vi "LangmuirProbe-V-I-processing.vi"() -> ()   [LabVIEW 2014]
uses:
  subvi/myInteger.ctl
  <vilib>/Utility/miscctls.llb/LVPositionTypeDef.ctl
  <vilib>/Analysis/baseanly.llb/Mean (DBL).vi
  <vilib>/Analysis/3filter.llb/Savitzky-Golay Filter (DBL).vi
  <vilib>/Waveform/WDTOps.llb/WDT Waveform Duration DBL.vi
  <vilib>/Utility/file.llb/Read From Spreadsheet File (string).vi
  <vilib>/Utility/file.llb/Write To Spreadsheet File (string).vi
  <vilib>/Waveform/WDTOps.llb/WDT Get Waveform Subset DBL.vi
  <vilib>/measure/mascope.llb/Amplitude and Levels 1 chan.vi
  <vilib>/measure/NI_MAPro.lvlib
  <vilib>/Analysis/NI_AALBase.lvlib
panel:
  in  "zero drift control":T1={"start zero, ms"=1.0, "duration of zero,ms"=1.0, "'0',\nms"=FALSE} {"start zero, ms" min=0.15000000000000002 max=74.85000000000001; "duration of zero,ms" min=0.15000000000000002 max=74.85000000000001}
  in  "Cursor":bool
  in  "data info template":T2={"data path"="", "ADCintercadr_s"=1.0, "data info"={"use or not *.info.txt?"=0, "probe name"="NaN", "signal type"="NaN", "Unit"="NaN", "variable"="NaN", "attenuation factor"=1.0, "amplification factor"=1.0, "extracoef#1"=1.0, "extracoef#2"=1.0, "U cascade, kV"="NaN", "probe area, cm2"=1.0, "plasma, a.m.u."=1.0}, "channel_name"="", "channels_in_file"=0}
  in  "Boolean":bool
  out "saw biasing,adc":dbl format="%.3g"
  in  "sinchrY":bool
  in  "legend":bool
  in  "X axis":u16(ring)=1 items=["index", "time"]
  in  "êÃö":dbl=625.0
  in  "Vsmooth":bool
  in  "polyn.order V":i32=1 min=1
  in  "side points V":i32=2 min=2
  in  "I smooth":bool
  in  "polynomial order I":i32=1 min=1
  in  "side points I":i32=2 min=2
  in  "data select":T4={"V"=1, "I"=1, " V - \"noise\""=0, "I - \"noise\""=0, "1\"0\""=0.0, "2\"0\""=0.0, "3\"0\""=0.0, "4\"0\""=0.0, "Numeric"=0, "Numeric 2"=0, "Numeric 3"=0, "Numeric 4"=0, "U-nois subtr."=FALSE, "I-nois subtr."=FALSE} {"4\"0\"" format="%.4g"; "3\"0\"" format="%.4f"; "2\"0\"" format="%.4f"; "1\"0\"" format="%.4f"; "I - \"noise\"" items=["***", "11_05_54#1\\11_11_08", "11_05_54#2\\11_11_08", "11_05_54#3\\11_11_08", "11_05_54#4\\11_11_08", "11_05_54#5\\11_11_08", "11_05_54#6\\11_11_08", "11_05_54#7\\11_11_08", "11_05_54#8\\11_11_08", "11_05_54#9\\11_11_08", "11_05_54#10\\11_11_08", "11_05_54#11\\11_11_08", "11_05_54#12\\11_11_08", "11_05_54#13\\11_11_08", "11_05_54#14\\11_11_08", "11_05_54#15\\11_11_08", "11_05_54#16\\11_11_08", "11_05_54#17\\11_11_08", "11_05_54#18\\11_11_08", "11_05_54#19\\11_11_08", "11_05_54#20\\11_11_08", "11_05_54#21\\11_11_08", "11_05_54#22\\11_11_08", "11_05_54#23\\11_11_08", "11_05_54#24\\11_11_08", "11_05_54#25\\11_11_08", "11_05_54#26\\11_11_08", "11_05_54#27\\11_11_08", "11_05_54#28\\11_11_08", "11_05_54#29\\11_11_08", "11_05_54#30\\11_11_08"]; "V - \"noise\"" items=["***", "11_05_54#1\\11_11_08", "11_05_54#2\\11_11_08", "11_05_54#3\\11_11_08", "11_05_54#4\\11_11_08", "11_05_54#5\\11_11_08", "11_05_54#6\\11_11_08", "11_05_54#7\\11_11_08", "11_05_54#8\\11_11_08", "11_05_54#9\\11_11_08", "11_05_54#10\\11_11_08", "11_05_54#11\\11_11_08", "11_05_54#12\\11_11_08", "11_05_54#13\\11_11_08", "11_05_54#14\\11_11_08", "11_05_54#15\\11_11_08", "11_05_54#16\\11_11_08", "11_05_54#17\\11_11_08", "11_05_54#18\\11_11_08", "11_05_54#19\\11_11_08", "11_05_54#20\\11_11_08", "11_05_54#21\\11_11_08", "11_05_54#22\\11_11_08", "11_05_54#23\\11_11_08", "11_05_54#24\\11_11_08", "11_05_54#25\\11_11_08", "11_05_54#26\\11_11_08", "11_05_54#27\\11_11_08", "11_05_54#28\\11_11_08", "11_05_54#29\\11_11_08", "11_05_54#30\\11_11_08"]; "I" items=["***", "11_05_54#1\\11_11_08", "11_05_54#2\\11_11_08", "11_05_54#3\\11_11_08", "11_05_54#4\\11_11_08", "11_05_54#5\\11_11_08", "11_05_54#6\\11_11_08", "11_05_54#7\\11_11_08", "11_05_54#8\\11_11_08", "11_05_54#9\\11_11_08", "11_05_54#10\\11_11_08", "11_05_54#11\\11_11_08", "11_05_54#12\\11_11_08", "11_05_54#13\\11_11_08", "11_05_54#14\\11_11_08", "11_05_54#15\\11_11_08", "11_05_54#16\\11_11_08", "11_05_54#17\\11_11_08", "11_05_54#18\\11_11_08", "11_05_54#19\\11_11_08", "11_05_54#20\\11_11_08", "11_05_54#21\\11_11_08", "11_05_54#22\\11_11_08", "11_05_54#23\\11_11_08", "11_05_54#24\\11_11_08", "11_05_54#25\\11_11_08", "11_05_54#26\\11_11_08", "11_05_54#27\\11_11_08", "11_05_54#28\\11_11_08", "11_05_54#29\\11_11_08", "11_05_54#30\\11_11_08"]; "V" items=["***", "11_05_54#1\\11_11_08", "11_05_54#2\\11_11_08", "11_05_54#3\\11_11_08", "11_05_54#4\\11_11_08", "11_05_54#5\\11_11_08", "11_05_54#6\\11_11_08", "11_05_54#7\\11_11_08", "11_05_54#8\\11_11_08", "11_05_54#9\\11_11_08", "11_05_54#10\\11_11_08", "11_05_54#11\\11_11_08", "11_05_54#12\\11_11_08", "11_05_54#13\\11_11_08", "11_05_54#14\\11_11_08", "11_05_54#15\\11_11_08", "11_05_54#16\\11_11_08", "11_05_54#17\\11_11_08", "11_05_54#18\\11_11_08", "11_05_54#19\\11_11_08", "11_05_54#20\\11_11_08", "11_05_54#21\\11_11_08", "11_05_54#22\\11_11_08", "11_05_54#23\\11_11_08", "11_05_54#24\\11_11_08", "11_05_54#25\\11_11_08", "11_05_54#26\\11_11_08", "11_05_54#27\\11_11_08", "11_05_54#28\\11_11_08", "11_05_54#29\\11_11_08", "11_05_54#30\\11_11_08"]}
  in  "plot color":T5={"color1"=43051, "color2"=393471, "color3"=13762815, "color4"=16722475}
  in  "cursor":bool
  in  "apply param.":bool
  out "Y":dbl=0.9225555555555554 format="%#.6f"
  out "X":dbl=0.04447201268742792 format="%#.7f"
  in  "param.input":bool
  in  "stop 2":bool
  in  "stop":bool
  out "data view":waveform(dbl)[](graph) caption="ADC data"
  in  "Tab Control":enum32{"Te&ne"}(tab)
  in  "show XY":bool
  in  "autoscale":bool=TRUE
  out "manual I-V source":string[][](table)=[["30", "-0.5118"], ["20", "0.38385"], ["10", "1.9619"], ["0", "2.60165"], ["-4", "2.3884"], ["-5", "2.8149"], ["-10", "2.85755"], ["-11", "3.19875"], ["-20", "3.2414"], ["-60", "4.05175"], ["-80", "4.1797"], ["-100", "3.96645"], ["-130", "4.265"]] caption="manual I-V inpu"
  in  "manual I-V input":string[][](table)=[["30", "-0.5118"], ["20", "0.38385"], ["10", "1.9619"], ["0", "2.60165"], ["-4", "2.3884"], ["-5", "2.8149"], ["-10", "2.85755"], ["-11", "3.19875"], ["-20", "3.2414"], ["-60", "4.05175"], ["-80", "4.1797"], ["-100", "3.96645"], ["-130", "4.265"]] caption="manual I-V inpu"
  in  "Fit scales":bool
  in  "show/hide table":bool
  in  "man. points":bool
  in  "del. points":bool
  in  "man.XY table":bool
  out "TeNe":cluster{cdb[]}[](graph)=[{[nan+0.474455i, nan+0.415499i, nan+0.873553i, 10.1+17.942145i, 10.3+20.809732i, 10.4+20.192076i, 10.7+20.192076i, 10.7+29.74605i, 10.7+24.903581i, 12.0+20.184913i, 12.0+1190171.81586i, 14.0+29.746054i]}, {[nan+48551830000.0i, nan+44679440000.0i, nan+41846650000.0i, 10.1+1606494000000.0i, 10.3+1406263000000.0i, 10.4+1449819000000.0i, 10.7+1288728000000.0i, 10.7+1769306000000.0i, 10.7+2116097000000.0i, 12.0+2004418000000.0i, 12.0+501530900000000.0i, 14.0+95067200000.0i]}]
  in  "manual coef. input":bool
  in  "manual param. input":T6={"R, ohm"=100.0, "saw bias., V"=180.0, "plasma, a.u.m."=1.0, "probe area, cm^2"=0.07, "position, etc."=13.999999999999996, "probe name"="VG8#1", "I amplif."=10.0, "saw bias., V(ADC)"=0.0} {"saw bias., V(ADC)" format="%#.6f"; "saw bias., V" min=1.0}
  in  "Limited by cursors":bool
  in  "Parameter Name      Parameter Guess        Fit?":T7={"parameter"="Te, eV", "Te_guess"=10.0, "Fit?"=TRUE} {"Te_guess" min=0.0}
  in  "Parameter Name      Parameter Guess        Fit? 3":T8={"parameter"="Vfl, V", "Vf_guess"=-10.0, "Fit?"=TRUE}
  in  "parameter                 manual            auto?":T9={"parameter"="Is, A", "Is_guess"=0.01, "Fit?"=TRUE}
  in  "save result":bool
  in  "processing":bool
  in  "show result":bool
  out "param.        manual.     auto?      auto             result":T10(array[cluster])=[{"parameter"="Is(mA)", "guess"=5.0, "Fit?"=TRUE, "best fit"=3.774695434023404, "result"=3.774695434023404}, {"parameter"="Vfl(V)", "guess"=0.0, "Fit?"=TRUE, "best fit"=-1.3923455769080333, "result"=-1.3923455769080333}, {"parameter"="Te(eV)", "guess"=3.0, "Fit?"=TRUE, "best fit"=1.9615172489090944, "result"=1.9615172489090944}] {"result" format="%#.6f"; "best fit" format="%#.6f"}
  out "density, cm^(-3)":dbl=24256512471.923824 format="%#.2e"
  out "Y":dbl format="%#.2g"
  out "X":dbl format="%#.2g"
  out "ln(I,I-bestfit)":cluster{cdb[]}[](graph)
  out "VI-fitgraph":cluster{cdb[]}[](graph)=[{[30.0-0.5118i, 20.0+0.38385i, 10.0+1.9619i, 0.0+2.60165i, -4.0+2.3884i, -5.0+2.8149i, -10.0+2.85755i, -11.0+3.19875i, -20.0+3.2414i, -60.0+4.05175i, -80.0+4.1797i, -100.0+3.96645i, -130.0+4.265i]}]
  out "result table":string[][](array[string])=[["                     file", "                 interval", "               probe name", "                 variable", "                  Is (mA)", "              Vfl (Volts)", "                  Te (eV)", "         density (cm**-3)"], ["                 10_36_46", "           t0.0373-0.0398", "                      NaN", "                      NaN", "                 3.715870", "                -0.124411", "                 0.474455", "             4.855183E+10"], ["                 10_10_55", "           t0.0152-0.0784", "                      NaN", "                      NaN", "                 3.200000", "                -0.087612", "                 0.415499", "             4.467944E+10"], ["                 10_12_10", "           t0.0272-0.0353", "                      NaN", "                      NaN", "                 4.345731", "                -0.052320", "                 0.873553", "             4.184665E+10"], ["                 10_45_04", "           t0.0235-0.0275", "                    VG8#1", "                10.100000", "                52.926325", "                -4.701742", "                17.942145", "             1.606494E+12"], ["                 10_45_04", "           t0.0235-0.0275", "                    VG8#1", "                10.300000", "                57.022652", "                -4.877215", "                20.809732", "             1.406263E+12"], ["                 10_45_04", "           t0.0235-0.0275", "                    VG8#1", "                10.400000", "                57.909756", "                -4.862004", "                20.192076", "             1.449819E+12"], ["                 10_45_04", "           t0.0235-0.0275", "                    VG8#1", "                10.700000", "                57.909756", "                -4.862004", "                20.192076", "             1.288728E+12"], ["                 10_45_04", "           t0.0235-0.0275", "                    VG8#1", "                10.700000", "                64.331903", "                -5.056201", "                29.746050", "             1.769306E+12"], ["                 10_45_04", "           t0.0235-0.0275", "                    VG8#1", "                10.700000", "                58.667018", "                -5.613754", "                24.903581", "             2.116097E+12"], ["                 10_45_04", "           t0.0235-0.0275", "                    VG8#1", "                12.000000", "                50.029859", "                -5.289460", "                20.184913", "             2.004418E+12"], ["                 10_45_04", "           t0.0235-0.0275", "                    VG8#1", "                12.000000", "           3039694.842475", "                -6.242550", "           1190171.815860", "             5.015309E+14"], ["                 10_45_04", "           t0.0235-0.0275", "                    VG8#1", "                14.000000", "                57.610661", "                -5.056201", "                29.746054", "             9.506720E+10"]]
  out "TeNe result":path=path "d:/_TeNe.txt"
  out "TeNe file":string="***"
  out "TeNe interval":string="t0.0216-0.0259"
  in  "press after parameters input":bool
  out "data info manual input sample":string[][](table)=[["11_00_19", "2", "VG1#1", "LP_biasing", "10.25", "1", "1", "162", "1", "5,6", "0.07", "1"], ["=", "4", "VG1#2", "LP_current", "10.25", "1", "1", "300", "1", "5,6", "0.07", "1"], ["11_00_44", "2", "VG1#1", "LP_biasing", "10.25", "1", "1", "162", "1", "5,6", "0.07", "1"], ["=", "4", "VG1#2", "LP_current", "10.25", "1", "1", "300", "1", "5,6", "0.07", "1"]]
  in  "data info manual input":string[][](table)=[["11_00_44", "2", "", "V", "10.25", "", "1", "162", "", "", "0.07", "1"], ["=", "4", "", "I", "10.25", "", "1", "300", "", "", "0.07", "1"], ["11_00_44", "2", "", "V", "10.25", "", "1", "162", "", "", "0.07", "1"], ["=", "4", "", "I", "10.25", "", "1", "300", "", "", "0.07", "1"], ["11_00_44", "2", "", "V", "10.25", "", "1", "162", "", "", "0.07", "1"], ["=", "4", "", "I", "10.25", "", "1", "300", "", "", "0.07", "1"]]
  out "source":T11={"data path"=["D:\\LCard\\ADC\\LPBPP\\30_09_15\\_0214_E-2010_4R235953#1", "D:\\LCard\\ADC\\LPBPP\\30_09_15\\_0214_E-2010_4R235953#2", "D:\\LCard\\ADC\\LPBPP\\30_09_15\\_0214_E-2010_4R235953#3"], "data"=[{"t0"=timestamp(0 s since 1904-01-01), "dt"=4e-07, "Y"=array[250000 elements], "attributes"=variant("info"=variant(cluster{"data path":string, "ADCcadrlength_s":dbl, "data info":cluster{"use or not *.info.txt?":i16, "probe name":string, "signal type":string, "Unit":string, "variable":string, "attenuation factor":dbl, "amplification factor":dbl, "extracoef#1":dbl, "extracoef#2":dbl, "U cascade, kV":string, "probe area, cm2":dbl, "plasma, a.m.u.":dbl}} {"data path"="D:\\LCard\\ADC\\LPBPP\\30_09_15\\_0214_E-2010_4R235953#1", "ADCcadrlength_s"=2500000.0, "data info"={"use or not *.info.txt?"=0, "probe name"="NaN", "signal type"="NaN", "Unit"="NaN", "variable"="NaN", "attenuation factor"=1.0, "amplification factor"=1.0, "extracoef#1"=1.0, "extracoef#2"=1.0, "U cascade, kV"="NaN", "probe area, cm2"=1.0, "plasma, a.m.u."=1.0}}))}, {"t0"=timestamp(1.3333333333330043e-07 s since 1904-01-01), "dt"=4e-07, "Y"=array[250000 elements], "attributes"=variant("info"=variant(cluster{"data path":string, "ADCcadrlength_s":dbl, "data info":cluster{"use or not *.info.txt?":i16, "probe name":string, "signal type":string, "Unit":string, "variable":string, "attenuation factor":dbl, "amplification factor":dbl, "extracoef#1":dbl, "extracoef#2":dbl, "U cascade, kV":string, "probe area, cm2":dbl, "plasma, a.m.u.":dbl}} {"data path"="D:\\LCard\\ADC\\LPBPP\\30_09_15\\_0214_E-2010_4R235953#2", "ADCcadrlength_s"=2500000.0, "data info"={"use or not *.info.txt?"=0, "probe name"="NaN", "signal type"="NaN", "Unit"="NaN", "variable"="NaN", "attenuation factor"=1.0, "amplification factor"=1.0, "extracoef#1"=1.0, "extracoef#2"=1.0, "U cascade, kV"="NaN", "probe area, cm2"=1.0, "plasma, a.m.u."=1.0}}))}, {"t0"=timestamp(2.666666666666551e-07 s since 1904-01-01), "dt"=4e-07, "Y"=array[250000 elements], "attributes"=variant("info"=variant(cluster{"data path":string, "ADCcadrlength_s":dbl, "data info":cluster{"use or not *.info.txt?":i16, "probe name":string, "signal type":string, "Unit":string, "variable":string, "attenuation factor":dbl, "amplification factor":dbl, "extracoef#1":dbl, "extracoef#2":dbl, "U cascade, kV":string, "probe area, cm2":dbl, "plasma, a.m.u.":dbl}} {"data path"="D:\\LCard\\ADC\\LPBPP\\30_09_15\\_0214_E-2010_4R235953#3", "ADCcadrlength_s"=2500000.0, "data info"={"use or not *.info.txt?"=0, "probe name"="NaN", "signal type"="NaN", "Unit"="NaN", "variable"="NaN", "attenuation factor"=1.0, "amplification factor"=1.0, "extracoef#1"=1.0, "extracoef#2"=1.0, "U cascade, kV"="NaN", "probe area, cm2"=1.0, "plasma, a.m.u."=1.0}}))}]}
  out "num-of-plots":i32=4
  out "data cut":T12={"data offset array"=[0.021598275434243176, 0.021598275434243176, 0.021598275434243176, 0.021598275434243176, 0.021598275434243176, 0.021598275434243176], "data cut array"=[{"t0"=timestamp(0.0215984 s since 1904-01-01), "dt"=4e-07, "Y"=array[10854 elements], "attributes"=variant("info"=variant(cluster{"data path":string, "ADCintercadr_s":dbl, "data info":cluster{"use or not *.info.txt?":i16, "probe name":string, "signal type":string, "Unit":string, "variable":string, "attenuation factor":dbl, "amplification factor":dbl, "extracoef#1":dbl, "extracoef#2":dbl, "U cascade, kV":string, "probe area, cm2":dbl, "plasma, a.m.u.":dbl}} {"data path"="***", "ADCintercadr_s"=2500000.0, "data info"={"use or not *.info.txt?"=0, "probe name"="NaN", "signal type"="NaN", "Unit"="NaN", "variable"="NaN", "attenuation factor"=1.0, "amplification factor"=1.0, "extracoef#1"=1.0, "extracoef#2"=1.0, "U cascade, kV"="NaN", "probe area, cm2"=1.0, "plasma, a.m.u."=1.0}}))}, {"t0"=timestamp(0.0215984 s since 1904-01-01), "dt"=4e-07, "Y"=array[10854 elements], "attributes"=variant("info"=variant(cluster{"data path":string, "ADCintercadr_s":dbl, "data info":cluster{"use or not *.info.txt?":i16, "probe name":string, "signal type":string, "Unit":string, "variable":string, "attenuation factor":dbl, "amplification factor":dbl, "extracoef#1":dbl, "extracoef#2":dbl, "U cascade, kV":string, "probe area, cm2":dbl, "plasma, a.m.u.":dbl}} {"data path"="***", "ADCintercadr_s"=2500000.0, "data info"={"use or not *.info.txt?"=0, "probe name"="NaN", "signal type"="NaN", "Unit"="NaN", "variable"="NaN", "attenuation factor"=1.0, "amplification factor"=1.0, "extracoef#1"=1.0, "extracoef#2"=1.0, "U cascade, kV"="NaN", "probe area, cm2"=1.0, "plasma, a.m.u."=1.0}}))}, {"t0"=timestamp(0.0215984 s since 1904-01-01), "dt"=4e-07, "Y"=array[10854 elements], "attributes"=variant("info"=variant(cluster{"data path":string, "ADCintercadr_s":dbl, "data info":cluster{"use or not *.info.txt?":i16, "probe name":string, "signal type":string, "Unit":string, "variable":string, "attenuation factor":dbl, "amplification factor":dbl, "extracoef#1":dbl, "extracoef#2":dbl, "U cascade, kV":string, "probe area, cm2":dbl, "plasma, a.m.u.":dbl}} {"data path"="***", "ADCintercadr_s"=2500000.0, "data info"={"use or not *.info.txt?"=0, "probe name"="NaN", "signal type"="NaN", "Unit"="NaN", "variable"="NaN", "attenuation factor"=1.0, "amplification factor"=1.0, "extracoef#1"=1.0, "extracoef#2"=1.0, "U cascade, kV"="NaN", "probe area, cm2"=1.0, "plasma, a.m.u."=1.0}}))}, {"t0"=timestamp(0.0215984 s since 1904-01-01), "dt"=4e-07, "Y"=array[10854 elements], "attributes"=variant("info"=variant(cluster{"data path":string, "ADCintercadr_s":dbl, "data info":cluster{"use or not *.info.txt?":i16, "probe name":string, "signal type":string, "Unit":string, "variable":string, "attenuation factor":dbl, "amplification factor":dbl, "extracoef#1":dbl, "extracoef#2":dbl, "U cascade, kV":string, "probe area, cm2":dbl, "plasma, a.m.u.":dbl}} {"data path"="***", "ADCintercadr_s"=2500000.0, "data info"={"use or not *.info.txt?"=0, "probe name"="NaN", "signal type"="NaN", "Unit"="NaN", "variable"="NaN", "attenuation factor"=1.0, "amplification factor"=1.0, "extracoef#1"=1.0, "extracoef#2"=1.0, "U cascade, kV"="NaN", "probe area, cm2"=1.0, "plasma, a.m.u."=1.0}}))}, {"t0"=timestamp(0.0215984 s since 1904-01-01), "dt"=4e-07, "Y"=array[10854 elements], "attributes"=variant("info"=variant(cluster{"data path":string, "ADCintercadr_s":dbl, "data info":cluster{"use or not *.info.txt?":i16, "probe name":string, "signal type":string, "Unit":string, "variable":string, "attenuation factor":dbl, "amplification factor":dbl, "extracoef#1":dbl, "extracoef#2":dbl, "U cascade, kV":string, "probe area, cm2":dbl, "plasma, a.m.u.":dbl}} {"data path"="***", "ADCintercadr_s"=2500000.0, "data info"={"use or not *.info.txt?"=0, "probe name"="NaN", "signal type"="NaN", "Unit"="NaN", "variable"="NaN", "attenuation factor"=1.0, "amplification factor"=1.0, "extracoef#1"=1.0, "extracoef#2"=1.0, "U cascade, kV"="NaN", "probe area, cm2"=1.0, "plasma, a.m.u."=1.0}}))}, {"t0"=timestamp(0.0215984 s since 1904-01-01), "dt"=4e-07, "Y"=array[10854 elements], "attributes"=variant("info"=variant(cluster{"data path":string, "ADCintercadr_s":dbl, "data info":cluster{"use or not *.info.txt?":i16, "probe name":string, "signal type":string, "Unit":string, "variable":string, "attenuation factor":dbl, "amplification factor":dbl, "extracoef#1":dbl, "extracoef#2":dbl, "U cascade, kV":string, "probe area, cm2":dbl, "plasma, a.m.u.":dbl}} {"data path"="***", "ADCintercadr_s"=2500000.0, "data info"={"use or not *.info.txt?"=0, "probe name"="NaN", "signal type"="NaN", "Unit"="NaN", "variable"="NaN", "attenuation factor"=1.0, "amplification factor"=1.0, "extracoef#1"=1.0, "extracoef#2"=1.0, "U cascade, kV"="NaN", "probe area, cm2"=1.0, "plasma, a.m.u."=1.0}}))}], "data lables"=["***=t0.0216-0.0259", "***=t0.0216-0.0259", "***=t0.0216-0.0259", "***=t0.0216-0.0259", "***=t0.0216-0.0259", "***=t0.0216-0.0259"], "short data lables"=["\\***=t0.0216-0.0259", "\\***=t0.0216-0.0259", "\\***=t0.0216-0.0259", "\\***=t0.0216-0.0259", "\\***=t0.0216-0.0259", "\\***=t0.0216-0.0259"]}
  # "ctr+\"click\" to add points !"
  # "set all parameters as close as possible\nto expected values !!!"
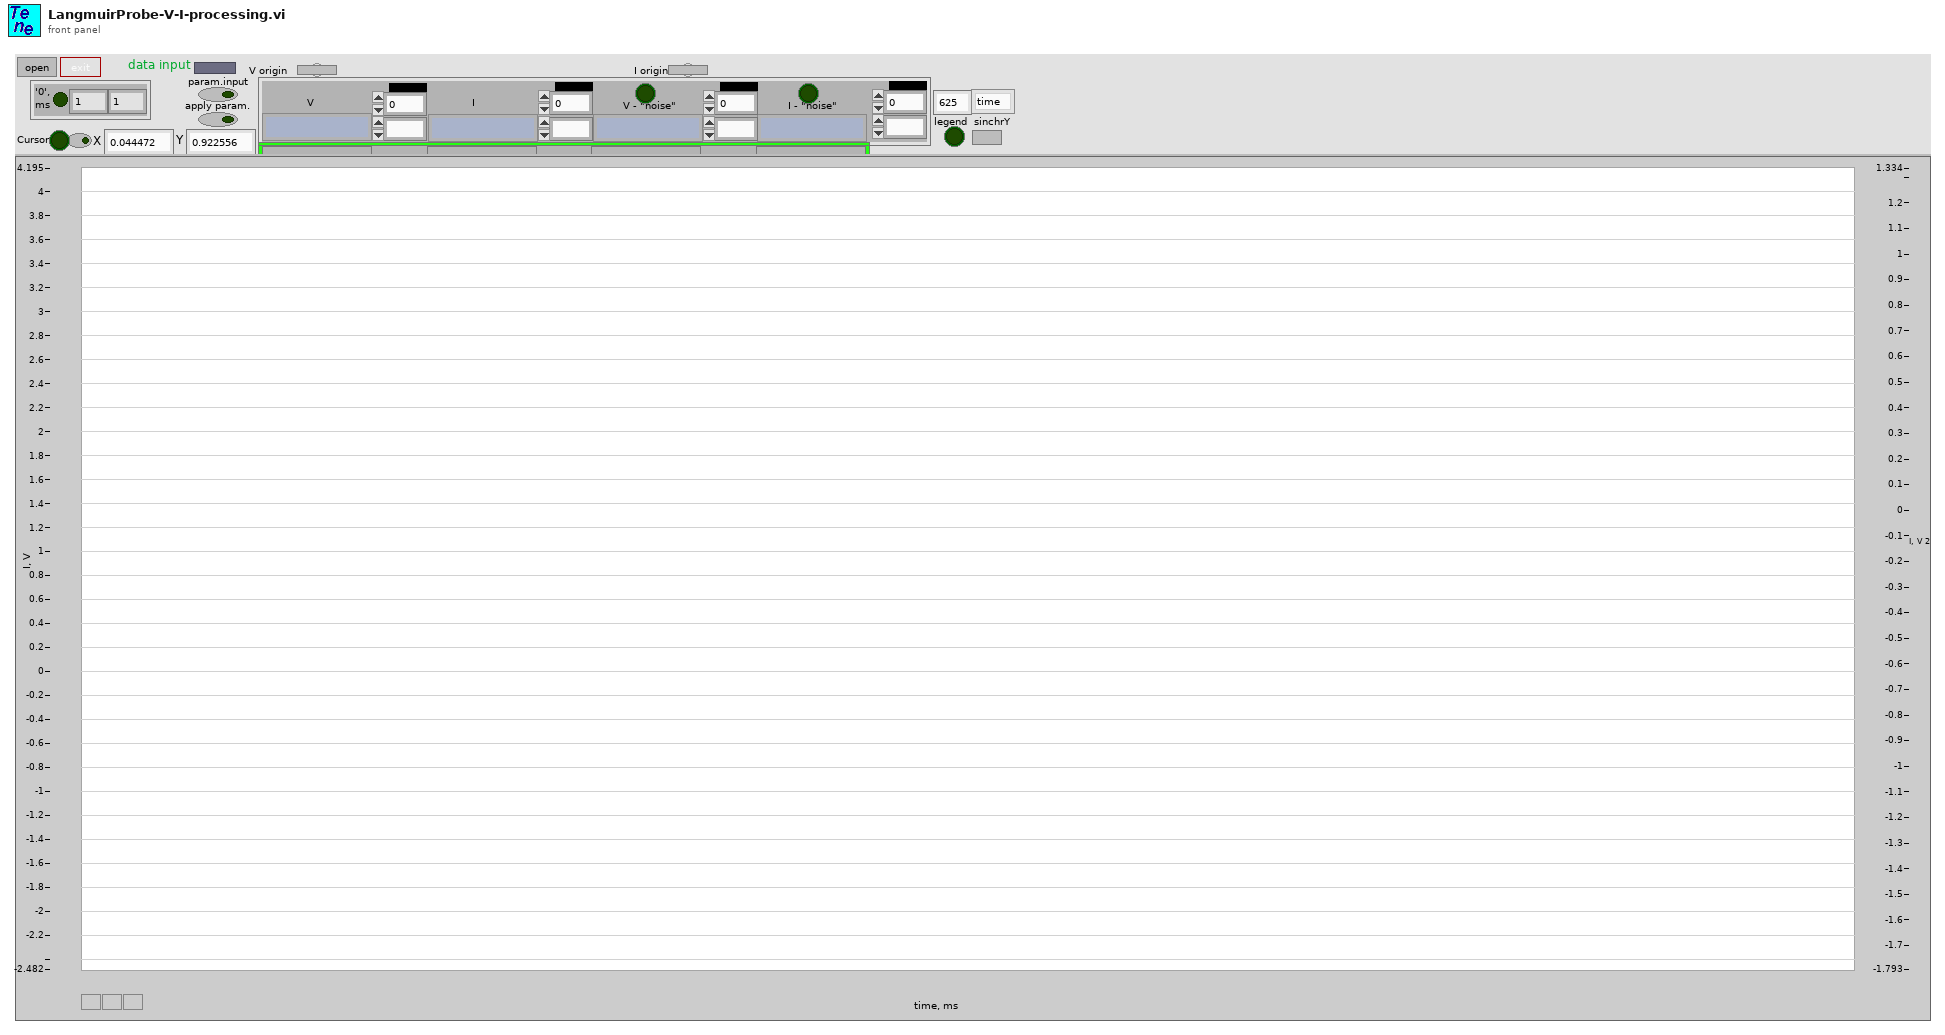
[diagram p1: front panel]
types:
  T1 = cluster{"start zero, ms":dbl, "duration of zero,ms":dbl, "'0',\nms":bool}
  T2 = cluster{"data path":string, "ADCintercadr_s":dbl, "data info":cluster{"use or not *.info.txt?":i16, "probe name":string, "signal type":string, "Unit":string, "variable":string, "attenuation factor":dbl, "amplification factor":dbl, "extracoef#1":dbl, "extracoef#2":dbl, "U cascade, kV":string, "probe area, cm2":dbl, "plasma, a.m.u.":dbl}, "channel_name":string, "channels_in_file":i32}
  T3 = typedef "myInteger.ctl" = i32
  T4 = cluster{"V":u16, "I":u16, " V - \"noise\"":u16, "I - \"noise\"":u16, "1\"0\"":dbl, "2\"0\"":dbl, "3\"0\"":dbl, "4\"0\"":dbl, "Numeric":T3, "Numeric 2":T3, "Numeric 3":T3, "Numeric 4":T3, "U-nois subtr.":bool, "I-nois subtr.":bool}
  T5 = cluster{"color1":u32, "color2":u32, "color3":u32, "color4":u32}
  T6 = cluster{"R, ohm":dbl, "saw bias., V":dbl, "plasma, a.u.m.":dbl, "probe area, cm^2":dbl, "position, etc.":dbl, "probe name":string, "I amplif.":dbl, "saw bias., V(ADC)":dbl}
  T7 = cluster{"parameter":string, "Te_guess":dbl, "Fit?":bool}
  T8 = cluster{"parameter":string, "Vf_guess":dbl, "Fit?":bool}
  T9 = cluster{"parameter":string, "Is_guess":dbl, "Fit?":bool}
  T10 = cluster{"parameter":string, "guess":dbl, "Fit?":bool, "best fit":dbl, "result":dbl}[]
  T11 = cluster{"data path":string[], "data":waveform(dbl)[]}
  T12 = cluster{"data offset array":dbl[], "data cut array":waveform(dbl)[], "data lables":string[], "short data lables":string[]}
  T13 = typedef "LVPositionTypeDef.ctl" = cluster{"Left":i32, "Top":i32}
  T14 = cluster{"method":enum32{"histogram", "peak", "auto select"}, "histogram size":i32, "histogram method":enum16{"mode"}, "reserved":dbl}
  T15 = cluster{"Name":string, "Color":u32, "Style":u8, "Point Style":u8, "Name Visible":bool, "Allow Drag":bool, "Cursor Mode":u32, "Plot":i32, "Index":i32, "Position":cluster{"X":dbl, "Y":dbl}, "X Scale":u32, "Y Scale":u32, "Watch Plots":i32[], "Watch All Plots":bool, "Plot Area":i32, "Label Offset":cluster{"X":dbl, "Y":dbl}}
  T16 = cluster{"V":u16, "I":u16, " V - \"noise\"":u16, "I - \"noise\"":u16}
  T17 = cluster{cluster{"V":u16, "I":u16, " V - \"noise\"":u16, "I - \"noise\"":u16}, "plot color":cluster{"color1":u32, "color2":u32, "color3":u32, "color4":u32}}
  T18 = typedef "LVRangeTypeDef.ctl" = cluster{"Minimum":dbl, "Maximum":dbl, "Increment":dbl, "Minor Increment":dbl, "Start":dbl}
  T19 = cluster{"use or not *.info.txt?":i16, "probe name":string, "signal type":string, "Unit":string, "variable":string, "attenuation factor":dbl, "amplification factor":dbl, "extracoef#1":dbl, "extracoef#2":dbl, "U cascade, kV":string, "probe area, cm2":dbl, "plasma, a.m.u.":dbl}
  T20 = typedef "LVPointDoubleTypeDef.ctl" = cluster{"Cursor X":dbl, "Cursor Y":dbl}
  T21 = typedef "LVCursorListTypeDef.ctl" = cluster{"Name":string, "Color":u32, "Style":u8, "Point Style":u8, "Name Visible":bool, "Allow Drag":bool, "Cursor Mode":u32, "Plot":i32, "Index":i32, "Position":cluster{"X":dbl, "Y":dbl}, "X Scale":u32, "Y Scale":u32, "Watch Plots":i32[], "Watch All Plots":bool, "Plot Area":i32, "Label Offset":cluster{"X":dbl, "Y":dbl}}[]
  T22 = enum8{"Enabled", "Disabled", "Disabled and Grayed Out"}
  T23 = cluster{"parameter":string, "guess":dbl, "Fit?":bool, "best fit":dbl, "result":dbl}
  T24 = typedef "LVPoint32TypeDef.ctl" = cluster{"Horizontal":i32, "Vertical":i32}
  T25 = cluster{"Shift":bool, "Ctrl":bool, "Alt":bool, "Cmd":bool, "Opt":bool}
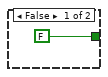
[diagram p3: hidden frame]
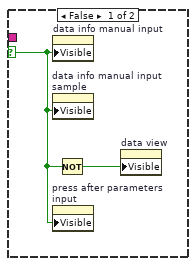
[diagram p5: hidden frame]
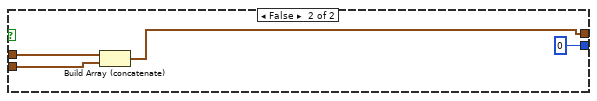
[diagram p9: hidden frame]
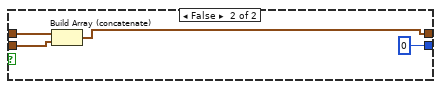
[diagram p10: hidden frame]
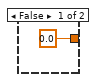
[diagram p11: hidden frame]
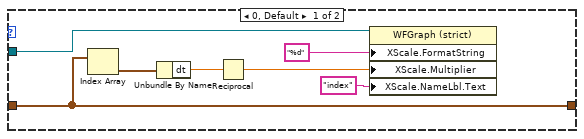
[diagram p13: hidden frame]
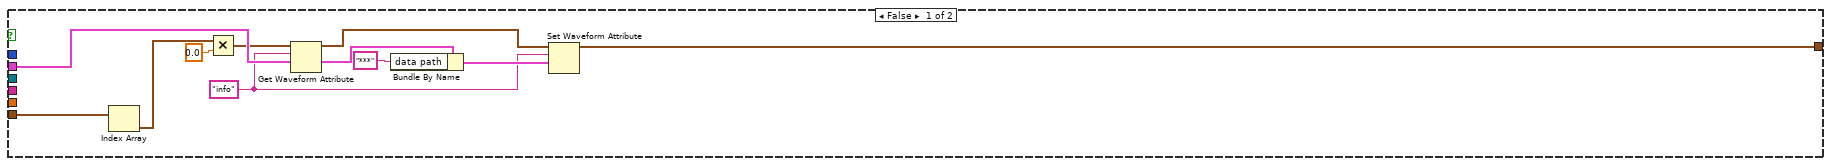
[diagram p14: hidden frame]
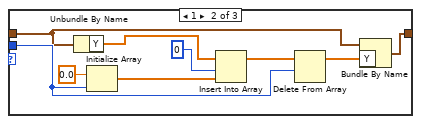
[diagram p16: hidden frame]
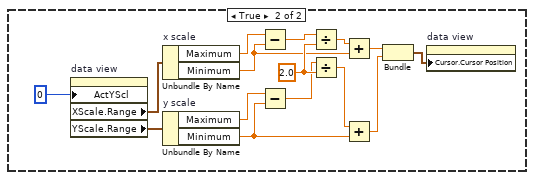
[diagram p18: hidden frame]
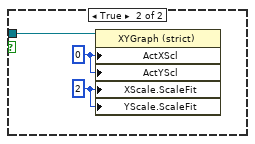
[diagram p20: hidden frame]
diagram:
  n1 = while {
    stop <- FALSE stop-if-true
    n2 = control-ref of="data info template"() -> (w5:refnum<vi>)
    n3 = call "DATAreader5.vi"("manual ADC rate, kHz"="êÃö", "data info template"=w5) -> ("error out"=w3:errorcluster, "source"=→"source":T11)  [unwired: 4 in, 4 out]
    n4 = invoke on="man.XY table" class="Bool (strict)" method="Reinit To Default"(error in=w3) -> (error out=w1:errorcluster)  [unwired: 2 in, 2 out]
    n5 = invoke on="processing" class="Bool (strict)" method="Reinit To Default"(error in=w1) -> (error out=w4:errorcluster)  [unwired: 2 in, 2 out]
    n6 = invoke on="Boolean" class="Bool (strict)" method="Reinit To Default"(error in=w4) -> (error out=w2:errorcluster)  [unwired: 2 in, 2 out]
    n7 = while {
      tunnel: w2 -> [w18]
      i -> [w12]
      stop <- "stop" stop-if-true
      n8 = control-ref of="data view"() -> (w9:refnum<vi>)
      n9 = Wait (ms)(milliseconds to wait=u32 300) -> ()  [unwired: 1 out]
      n10 = case shown="True" "Boolean" {
        tunnel: w18 -> [w35 _]
        frame False {
          n11 = flat-sequence {
            tunnel: w35 -> [w62]
            tunnel: [w62] -> w33
            tunnel: [w37] -> w31
            tunnel: [w60] -> w29
            tunnel: [w57] -> w27
            tunnel: w33 -> [w75]
            tunnel: [w75] -> w32
            tunnel: w31 -> [w74]
            tunnel: [w74] -> w30
            tunnel: w29 -> [w72]
            tunnel: [w72] -> w28
            tunnel: w27 -> [w73]
            tunnel: [w73] -> w26
            tunnel: w32 -> [_]
            tunnel: w30 -> [w156]
            tunnel: w28 -> [w155]
            tunnel: w26 -> [w154]
            tunnel: [w135] -> w23
            tunnel: [w299] -> w24
            tunnel: w23 -> [w299]
            tunnel: w24 -> [w327]
            frame #0 {
              w42 = u8 1 ("Response to Value Outside Limits:Maximum")
              w43 = 1000.0 ("y")
              n12 = local read "source"() -> (w61:T11)
              n13 = property on="Splitter" class="Splitter"("Position"=100 ("Splitter Position")) -> ()  [unwired: 2 in, 2 out]
              n14 = Unbundle By Name(w61) -> ("data path"=w60:string[], "data"=w37:waveform(dbl)[])
              n15 = for {
                tunnel: w60 -> [w70] mode=indexing
                tunnel: [w66] -> w58 mode=indexing
                w65 = "\\" ("regular expression")
                n16 = Reverse String(1:w70) -> (0:w69:string)
                n17 = Match Pattern(string=w69, regular expression=w65) -> (before substring=w63:string, after substring=w68:string)  [unwired: 1 in, 2 out]
                n18 = Match Pattern(string=w68, regular expression=w65) -> (before substring=w64:string)  [unwired: 1 in, 3 out]
                n19 = Concatenate Strings(w64, w65, w63) -> (w67:string)
                n20 = Reverse String(1:w67) -> (0:w66:string)
              }
              n21 = Index Array(array=w37) -> (element=w36:waveform(dbl))  [unwired: 1 in]
              n22 = call-poly <vilib>:"Waveform Duration.vi"("waveform in"=w36) -> ("duration"=w40:dbl, "waveform out"=w44:waveform(dbl))  [unwired: 8 in, 1 out]
              n23 = Unbundle By Name(w44) -> ("dt"=w41:dbl)
              n24 = Multiply(x=w41, y=w43) -> (x*y=w39:dbl)
              n25 = Multiply(x=w40, y=w43) -> (x*y=w38:dbl)
              n26 = property on="start zero, ms" class="DigNum (strict)"("Maximum"=w38, "Minimum"=w39, "OutOfRngActMax"=w42, "OutOfRngActMin"=w42) -> ()  [unwired: 2 in, 2 out]
              n27 = property on="duration of zero,ms" class="DigNum (strict)"("Maximum"=w38, "Minimum"=w39, "OutOfRngActMax"=w42, "OutOfRngActMin"=w42) -> ()  [unwired: 2 in, 2 out]
              n28 = Unbundle By Name("data select") -> ("V"=w50:u16, "I"=w49:u16, "V - \"noise\""=w48:u16, "I - \"noise\""=w47:u16)
              n29 = Bundle("V"=w50, "I"=w49, "V - \"noise\""=w48, "I - \"noise\""=w47) -> (w46:T16)  [unwired: 1 in]
              n30 = control-ref of="data view"() -> (w52:refnum<vi>)
              n31 = Build Array (concatenate)("***", w58) -> (w54:string[])
              n32 = Bundle(w46, "plot color"="plot color") -> (w55:T17)  [unwired: 1 in]
              n33 = property on="V" class="Ring (strict)"("Strings []"=w54) -> ()  [unwired: 2 in, 2 out]
              n34 = property on="I" class="Ring (strict)"("Strings []"=w54) -> ()  [unwired: 2 in, 2 out]
              n35 = property on="I - \"noise\"" class="Ring (strict)"("Strings []"=w54) -> ()  [unwired: 2 in, 2 out]
              n36 = property on="V - \"noise\"" class="Ring (strict)"("Strings []"=w54) -> ()  [unwired: 2 in, 2 out]
              n37 = call "plot_selector2.vi"("LegendON"="legend", "data lables"=w54, "selector"=w55, "cut data"=w52) -> ("data #"=w57:i32[])  [unwired: 3 in, 1 out]
            }
            frame #1 {
              n38 = case shown="True" "param.input" {
                selector: "param.input" -> [w76 w93]
                tunnel: w72 -> [_ w81]
                frame False {
                  n39 = property on="data info manual input" class="Tbl (strict)"("Visible"=w76) -> ()  [unwired: 2 in, 2 out]
                  n40 = property on="data info manual input sample" class="Tbl (strict)"("Visible"=w76) -> ()  [unwired: 2 in, 2 out]
                  n41 = property on="press after parameters input" class="Bool"("Visible"=w76) -> ()  [unwired: 2 in, 2 out]
                  n42 = Not(x=w76) -> (.not. x?=w77:bool)
                  n43 = property on="data view" class="WFGraph (strict)"("Visible"=w77) -> ()  [unwired: 2 in, 2 out]
                }
                frame True {
                  n44 = property on="press after parameters input" class="Bool"("Visible"=w93) -> ()  [unwired: 2 in, 2 out]
                  n45 = property on="data info manual input sample" class="Tbl (strict)"("Visible"=w93) -> ()  [unwired: 2 in, 2 out]
                  n46 = property on="data info manual input" class="Tbl (strict)"("Visible"=w93) -> ()  [unwired: 2 in, 2 out]
                  n47 = Index Array(array=w81) -> (element=w80:string)  [unwired: 1 in]
                  n48 = Not(x=w93) -> (.not. x?=w95:bool)
                  n49 = property on="data info manual input" class="Tbl (strict)"("Position"=T13 {"Left"=-2055, "Top"=272}) -> ()  [unwired: 2 in, 2 out]
                  n50 = property on="Splitter" class="Splitter"("Position"=22 ("Splitter Position")) -> ()  [unwired: 2 in, 2 out]
                  n51 = property on="data view" class="WFGraph (strict)"("Visible"=w95) -> ()  [unwired: 2 in, 2 out]
                  n52 = property on="data info manual input sample" class="Tbl (strict)"("Position"=T13 {"Left"=-2055, "Top"=155}) -> ()  [unwired: 2 in, 2 out]
                  n53 = property on="press after parameters input" class="Bool"("Position"=T13 {"Left"=-2000, "Top"=700}) -> ()  [unwired: 2 in, 2 out]
                  n54 = String To Path(string=w80) -> (path=w89:path)
                  n55 = Strip Path(path=w89) -> (stripped path=w84:path)  [unwired: 1 out]
                  n56 = Strip Path(path=w84) -> (name=w85:string)  [unwired: 1 out]
                  n57 = Concatenate Strings(w85, ".info.txt" ("string")) -> (w87:string)
                  n58 = Build Path(base path=w84, name or relative path=w87) -> (appended path=w86:path)
                  n59 = call <vilib>:"Check if File or Folder Exists.vi"("path"=w86) -> ("file or folder exists?"=w82:bool, "dup path"=w83:path)  [unwired: 8 in, 1 out]
                  n60 = flat-sequence {
                    tunnel: w83 -> [w98]
                    tunnel: [w97] -> w90
                    tunnel: w82 -> [w99]
                    tunnel: w90 -> [w104]
                    tunnel: [w105] -> w79
                    tunnel: [w104] -> w78
                    tunnel: w79 -> [w108]
                    tunnel: w78 -> [w109]
                    frame #0 {
                      n61 = case shown="True" w99 {
                        tunnel: w98 -> [w100 w103]
                        tunnel: [w100 w102] -> w97
                        frame False {
                        }
                        frame True {
                          n62 = call-poly <vilib>:"Read From Spreadsheet File.vi"("file path (dialog if empty)"=w103) -> ("all rows"=w101:string[][], "new file path (Not A Path if cancelled)"=w102:path)  [unwired: 6 in, 3 out]
                          n63 = property on="data info manual input" class="Tbl (strict)"("Value"=w101) -> ()  [unwired: 2 in, 2 out]
                        }
                      }
                    }
                    frame #1 {
                      n64 = while {
                        tunnel: ["data info manual input"] -> w105
                        stop <- "press after parameters input" stop-if-true
                      }
                    }
                    frame #2 {
                      n65 = call-poly <vilib>:"Write To Spreadsheet File.vi"("2D data"=w108, "file path (dialog if empty)"=w109) -> ()  [unwired: 6 in, 1 out]
                    }
                  }
                }
              }
            }
            frame #2 {
              n66 = local read "data select"() -> (w134:T4)
              n67 = case shown="True" "sinchrY" {
                frame False {
                }
                frame True {
                  n68 = property on="data view" class="WFGraph (strict)"("ActYScl"=0 ("Active Y Scale")) -> ("YScale.Range"=w157:T18)  [unwired: 2 in, 2 out]
                  n69 = property on="data view" class="WFGraph (strict)"("ActYScl"=1 ("Active Y Scale"), "YScale.Range"=w157) -> ()  [unwired: 2 in, 2 out]
                }
              }
              n70 = control-ref of="data info template"() -> (w117:refnum<vi>)
              n71 = Unbundle(w134) -> ("1\"0\""=w133:dbl, "2\"0\""=w132:dbl, "3\"0\""=w131:dbl, "4\"0\""=w130:dbl, "Numeric"=w128:T3, "Numeric 2"=w127:T3, "Numeric 3"=w126:T3, "Numeric 4"=w125:T3, "U-nois subtr."=w123:bool, "I-nois subtr."=w122:bool)  [unwired: 4 out]
              n72 = property class="Clust (strict)"(reference=w117) -> (reference out=w116:refnum<vi>, "Value"=w115:T2)  [unwired: 1 in, 1 out]
              n73 = Build Array(w133, w132, w131, w130) -> (w129:dbl[])
              n74 = Build Array(w128, w127, w126, w125) -> (w124:T3[])
              n75 = for {
                N -> [w222]
                tunnel: w154 -> [w221] mode=indexing
                tunnel: w156 -> [w223]
                tunnel: w155 -> [w224]
                tunnel: [w213] -> w149 mode=indexing
                tunnel: w129 -> [w218] mode=indexing
                tunnel: w124 -> [w217] mode=indexing
                tunnel: w117 -> [w215]
                tunnel: w115 -> [w214]
                n76 = To Long Integer(number=w217) -> (32bit integer=w216:T3)
                n77 = Not Equal?(x=w221, y=0) -> (x != y?=w219:bool)
                n78 = case shown="True" w219 {
                  tunnel: w224 -> [_ w269]
                  tunnel: w223 -> [w235 w268]
                  tunnel: w221 -> [_ w265]
                  tunnel: [w225 w255] -> w213
                  tunnel: w214 -> [w230 w257]
                  tunnel: w218 -> [_ w256]
                  tunnel: w216 -> [_ w246]
                  tunnel: w215 -> [_ w245]
                  frame False {
                    w229 = "info" ("name")
                    n79 = Index Array(array=w235) -> (element=w234:waveform(dbl))  [unwired: 1 in]
                    n80 = Multiply(x=w234, y=0.0) -> (x*y=w226:waveform(dbl))
                    n81 = Get Waveform Attribute(5:w230, 6:w229, 7:w226) -> (1:w228:T2, 3:w232:waveform(dbl))  [unwired: 1 in, 2 out]
                    n82 = Bundle By Name(cluster=w228, "data path"="***") -> (w231:T2)
                    n83 = Set Waveform Attribute(5:w231, 6:w229, 7:w232) -> (3:w225:waveform(dbl))  [unwired: 1 in, 2 out]
                  }
                  frame True {
                    w241 = 1000.0 ("y")
                    w261 = "info" ("name")
                    n84 = Absolute Value(x=w246) -> (abs(x)=w247:T3)
                    n85 = Greater Than 0?(x=w246) -> (x > 0?=w250:bool)
                    n86 = Decrement(x=w265) -> (x-1=w264:i32)
                    n87 = Index Array(array=w269, index=w264) -> (element=w266:string)
                    n88 = Index Array(array=w268, index=w264) -> (element=w267:waveform(dbl))
                    n89 = Equal To 0?(x=w246) -> (x = 0?=w254:bool)
                    n90 = Select(t=1, s=w250, f=2) -> (s? t:f=w251:i32)
                    n91 = call "InfoRead4.vi"("data info template"=w245, "source path"=w266) -> ("data from *.info.txt"=w258:T19)  [unwired: 3 in]
                    n92 = Select(t=0, s=w254, f=w251) -> (s? t:f=w252:i32)
                    n93 = Get Waveform Attribute(5:w257, 6:w261, 7:w267) -> (1:w260:T2, 3:w262:waveform(dbl))  [unwired: 1 in, 2 out]
                    n94 = Bundle By Name(cluster=w260, "data info"=w258) -> (w259:T2)
                    n95 = Unbundle By Name("zero drift control") -> ("start zero, ms"=w240:dbl, "duration of zero,ms"=w243:dbl, "'0',\nms"=w238:bool)
                    n96 = Set Waveform Attribute(5:w259, 6:w261, 7:w262) -> (3:w263:waveform(dbl))  [unwired: 1 in, 2 out]
                    n97 = Divide(x=w240, y=w241) -> (x/y=w242:dbl)
                    n98 = Divide(x=w243, y=w241) -> (x/y=w244:dbl)
                    n99 = Subtract(x=w263, y=w256) -> (x-y=w237:waveform(dbl))
                    n100 = case shown="True" w238 {
                      tunnel: w237 -> [w270 w274]
                      tunnel: [w270 w273] -> w236
                      tunnel: w242 -> [_ w276]
                      tunnel: w244 -> [_ w275]
                      frame False {
                      }
                      frame True {
                        w271 = u16 1 items=["Samples", "Relative Time"] ("start/duration format")
                        n101 = call-poly <vilib>:"Get Waveform Subset.vi"("start/duration format"=w271, "duration"=w275, "start samples/time"=w276, "waveform in"=w274) -> ("waveform out"=w277:waveform(dbl))  [unwired: 2 in, 3 out]
                        n102 = Unbundle By Name(w277) -> ("Y"=w278:dbl[])
                        n103 = call-poly <vilib>:"Mean.vi"("X"=w278) -> ("mean"=w272:dbl)  [unwired: 1 out]
                        n104 = Subtract(x=w274, y=w272) -> (x-y=w273:waveform(dbl))
                      }
                    }
                    n105 = case shown="2" w252 {
                      tunnel: [w279 w296 w297] -> w255
                      tunnel: w247 -> [w281 w294 _]
                      tunnel: w236 -> [w283 w292 w297]
                      frame 2 {
                        n106 = Unbundle By Name(w283) -> ("Y"=w280:dbl[])
                        n107 = Initialize Array(0.0 ("element"), w281) -> (w286:dbl[])
                        n108 = Insert Into Array(array=w280, new element=w286) -> (w285:dbl[])  [unwired: 1 in]
                        n109 = Delete From Array(array=w285, length=w281, index=0) -> (array with subset deleted=w287:dbl[])  [unwired: 1 out]
                        n110 = Bundle By Name(cluster=w283, "Y"=w287) -> (w279:waveform(dbl))
                      }
                      frame 1 {
                        n111 = Unbundle By Name(w292) -> ("Y"=w295:dbl[])
                        n112 = Initialize Array(0.0 ("element"), w294) -> (w291:dbl[])
                        n113 = Insert Into Array(array=w295, index=0, new element=w291) -> (w290:dbl[])
                        n114 = Delete From Array(array=w290, length=w294) -> (array with subset deleted=w293:dbl[])  [unwired: 1 in, 1 out]
                        n115 = Bundle By Name(cluster=w292, "Y"=w293) -> (w296:waveform(dbl))
                      }
                      frame 0, Default {
                      }
                    }
                  }
                }
                "num-of-plots" <- w222
              }
              n116 = control-ref of="data view"() -> (w152:refnum<vi>)
              n117 = local read "X axis"() -> (w153:u16)
              n118 = case "x-axis scaling" shown="1" w153 {
                tunnel: w152 -> [w207 w211]
                tunnel: w149 -> [w206 w210]
                tunnel: [w206 w210] -> w151
                frame 0, Default {
                  n119 = Index Array(array=w206) -> (element=w205:waveform(dbl))  [unwired: 1 in]
                  n120 = Unbundle By Name(w205) -> ("dt"=w204:dbl)
                  n121 = Reciprocal(x=w204) -> (1/x=w203:dbl)
                  n122 = property on="Property Node" class="WFGraph (strict)"(reference=w207, "XScale.FormatString"="%d" ("X Scale.Format String"), "XScale.Multiplier"=w203, "XScale.NameLbl.Text"="index" ("X Scale.Name Label.Text")) -> ()  [unwired: 1 in, 2 out]
                }
                frame 1 {
                  n123 = property on="Property Node" class="WFGraph (strict)"(reference=w211, "XScale.FormatString"="%#.6f" ("X Scale.Format String"), "XScale.Multiplier"=1000.0 ("X Scale.Offset and Multiplier:Multiplier"), "XScale.NameLbl.Text"="time, ms" ("X Scale.Name Label.Text")) -> ()  [unwired: 1 in, 2 out]
                }
              }
              n124 = call "removeU-Inois.vi"("I-nois subtr."=w122, "U-nois subtr."=w123, "Array in"=w151, "data info template"=w116) -> ("Array out"=w148:waveform(dbl)[])  [unwired: 7 in]
              n125 = case shown="True" "apply param." {
                tunnel: w148 -> [w197 w200]
                tunnel: [w197 w199] -> w112
                tunnel: w115 -> [_ w198]
                frame False {
                }
                frame True {
                  n126 = call "Normaliz3.1.vi"("data info template"=w198, "Array in"=w200) -> ("Array out"=w199:waveform(dbl)[])  [unwired: 9 in]
                }
              }
              n127 = Index Array "V"(array=w112) -> (element=w114:waveform(dbl))  [unwired: 1 in]
              n128 = case shown="True" "Vsmooth" {
                tunnel: w112 -> [w188 w192]
                tunnel: [w187 w191] -> w111
                tunnel: w114 -> [w180 w190]
                tunnel: [w178 0 ("error")] -> w139
                frame True {
                  n129 = call-poly <vilib>:"Savitzky-Golay Filter.vi"("polynomial order"="polyn.order V", "side points"="side points V", "X"=w180) -> ("error"=w178:i32, "Filtered X"=w184:dbl[])  [unwired: 7 in]
                  n130 = Bundle By Name(cluster=w180, "Y"=w184) -> (w179:waveform(dbl))
                  n131 = Set Waveform Attribute(5:"voltage best fit", 6:"NI_LineNames" ("name"), 7:w179) -> (3:w181:waveform(dbl))  [unwired: 1 in, 2 out]
                  n132 = Build Array (concatenate)(w188, w181) -> (w187:waveform(dbl)[])
                }
                frame False {
                  n133 = Build Array (concatenate)(w192, w190) -> (w191:waveform(dbl)[])
                }
              }
              n134 = property on="side points V" class="DigNum (strict)"("Visible"="Vsmooth") -> ()  [unwired: 2 in, 2 out]
              n135 = property on="polyn.order V" class="DigNum (strict)"("Visible"="Vsmooth") -> ()  [unwired: 2 in, 2 out]
              n136 = Index Array "V"(array=w111, index=4) -> (element=w110:waveform(dbl))
              n137 = Index Array "I"(array=w111, index=1) -> (element=w137:waveform(dbl))
              n138 = property on="side points I" class="DigNum (strict)"("Visible"="I smooth") -> ()  [unwired: 2 in, 2 out]
              n139 = property on="polynomial order I" class="DigNum (strict)"("Visible"="I smooth") -> ()  [unwired: 2 in, 2 out]
              n140 = case shown="True" "I smooth" {
                tunnel: w111 -> [w173 w177]
                tunnel: [w172 w176] -> w138
                tunnel: w137 -> [w167 w175]
                tunnel: [w163 0 ("error")] -> w140
                frame True {
                  n141 = call-poly <vilib>:"Savitzky-Golay Filter.vi"("polynomial order"="polynomial order I", "side points"="side points I", "X"=w167) -> ("error"=w163:i32, "Filtered X"=w171:dbl[])  [unwired: 7 in]
                  n142 = Bundle By Name(cluster=w167, "Y"=w171) -> (w166:waveform(dbl))
                  n143 = Set Waveform Attribute(5:"voltage best fit", 6:"NI_LineNames" ("name"), 7:w166) -> (3:w168:waveform(dbl))  [unwired: 1 in, 2 out]
                  n144 = Build Array (concatenate)(w173, w168) -> (w172:waveform(dbl)[])
                }
                frame False {
                  n145 = Build Array (concatenate)(w177, w175) -> (w176:waveform(dbl)[])
                }
              }
              n146 = Build Array (concatenate)(w112, w114, w137) -> (w136:waveform(dbl)[])
              n147 = call-poly <vilib>:"Amplitude and Levels.vi"("state settings"=T14 {"method"=enum."peak", "histogram size"=256, "histogram method"=enum."mode", "reserved"=1.0}, "signal in"=w110) -> ("amplitude"=w118:dbl)  [unwired: 6 in, 3 out]
              n148 = Not Equal To 0?(x=w118) -> (x != 0?=w120:bool)
              n149 = case shown="True" w120 {
                tunnel: w110 -> [_ w196]
                tunnel: [0.0 w194] -> w147
                frame False {
                }
                frame True {
                  n150 = call-poly <vilib>:"Amplitude and Levels.vi"("state settings"=T14 {"method"=enum."auto select", "histogram size"=256, "histogram method"=enum."mode", "reserved"=1.0}, "signal in"=w196) -> ("low state level"=w194:dbl)  [unwired: 6 in, 3 out]
                }
              }
              "saw biasing,adc" <- w147
              n151 = Not Equal To 0?(x=w140) -> (x != 0?=w143:bool)
              n152 = Not Equal To 0?(x=w139) -> (x != 0?=w142:bool)
              n153 = Or(x=w143, y=w142) -> (x .or. y?=w141:bool)
              n154 = case shown="True" w141 {
                tunnel: [w160 w161] -> w135
                tunnel: w138 -> [w160 _]
                tunnel: w136 -> [_ w161]
                frame False {
                }
                frame True {
                  w162 = 2
                  n155 = property on="polyn.order V" class="DigNum (strict)"("Value"=w162) -> ()  [unwired: 2 in, 2 out]
                  n156 = property on="polynomial order I" class="DigNum (strict)"("Value"=w162) -> ()  [unwired: 2 in, 2 out]
                  n157 = property on="side points I" class="DigNum (strict)"("Value"=w162) -> ()  [unwired: 2 in, 2 out]
                  n158 = property on="side points V" class="DigNum (strict)"("Value"=w162) -> ()  [unwired: 2 in, 2 out]
                }
              }
              "data view" <- w135
            }
            frame #3 {
              n159 = case shown="False" "cursor" {
                frame False {
                  n160 = property on="data view" class="WFGraph (strict)"("Active Cursor"=u32 0, "Cursor.Visible"="Cursor") -> ("Cursor.Cursor Position"=w302:T20)  [unwired: 2 in, 2 out]
                  n161 = Unbundle By Name(w302) -> ("Cursor X"=→"X":dbl, "Cursor Y"=→"Y":dbl)
                }
                frame True {
                  w314 = 2.0 ("y")
                  n162 = property on="data view" class="WFGraph (strict)"("ActYScl"=0 ("Active Y Scale")) -> ("XScale.Range"=w319:T18, "YScale.Range"=w318:T18)  [unwired: 2 in, 2 out]
                  n163 = Unbundle By Name "x scale"(w319) -> ("Maximum"=w317:dbl, "Minimum"=w311:dbl)
                  n164 = Unbundle By Name "y scale"(w318) -> ("Maximum"=w316:dbl, "Minimum"=w309:dbl)
                  n165 = Subtract(x=w317, y=w311) -> (x-y=w315:dbl)
                  n166 = Subtract(x=w316, y=w309) -> (x-y=w313:dbl)
                  n167 = Divide(x=w315, y=w314) -> (x/y=w312:dbl)
                  n168 = Divide(x=w313, y=w314) -> (x/y=w310:dbl)
                  n169 = Add(x=w312, y=w311) -> (x+y=w308:dbl)
                  n170 = Add(x=w310, y=w309) -> (x+y=w307:dbl)
                  n171 = Bundle(w308, w307) -> (w306:cluster{dbl, dbl})  [unwired: 1 in]
                  n172 = property on="data view" class="WFGraph (strict)"("Cursor.Cursor Position"=w306) -> ()  [unwired: 2 in, 2 out]
                }
              }
            }
            frame #4 {
              n173 = property on="data view" class="WFGraph (strict)"() -> ("XScale.Range"=w328:T18)  [unwired: 2 in, 2 out]
              n174 = Unbundle By Name(w328) -> ("Minimum"=w323:dbl, "Maximum"=w324:dbl)
              n175 = local read "X axis"() -> (w325:u16)
              n176 = case shown="1" w325 {
                tunnel: w324 -> [w335 w340]
                tunnel: w323 -> [w334 w338]
                tunnel: [w335 w339] -> w320
                tunnel: [w334 w336] -> w322
                frame 0, Default {
                }
                frame 1 {
                  w337 = 1000.0 ("y")
                  n177 = Divide(x=w338, y=w337) -> (x/y=w336:dbl)
                  n178 = Divide(x=w340, y=w337) -> (x/y=w339:dbl)
                }
              }
              n179 = control-ref of="data info template"() -> (w321:refnum<vi>)
              n180 = for {
                tunnel: w325 -> [w349]
                tunnel: [w345] -> w326 mode=indexing
                tunnel: w322 -> [w344]
                tunnel: w320 -> [w346]
                tunnel: w327 -> [w351]
                tunnel: [w348] -> w331 mode=indexing
                tunnel: [w347] -> w330 mode=indexing
                tunnel: [w344] -> w329 mode=indexing
                tunnel: w327 -> [_] mode=indexing
                tunnel: w321 -> [w341]
                i -> [w343]
                n181 = Index Array(array=w351, index=w343) -> (element=w342:waveform(dbl))
                n182 = call "cut.vi"("start/duration format"=w349, "data info template"=w341, "input"=w342, "open interval? (T)"=TRUE, "cut  end"=w346, "Begin offset"=w344) -> ("Part of input"=w345:waveform(dbl), "short cut data lables"=w347:string, "cut data lables"=w348:string)
              }
              n183 = Bundle By Name(cluster=T12 {"data offset array"=[], "data cut array"=[], "data lables"=[], "short data lables"=[]} ("output cluster"), "data cut array"=w326, "data lables"=w331, "short data lables"=w330, "data offset array"=w329) -> (→"data cut":T12)
            }
          }
          n184 = property on="Tab Control" class="TabCtl (strict)"("Visible"=FALSE) -> ()  [unwired: 2 in, 2 out]
          n185 = property on="data view" class="WFGraph (strict)"("Visible"=TRUE) -> ()  [unwired: 2 in, 2 out]
        }
        frame True {
          n186 = flat-sequence {
            frame #0 {
              w437 = u16 5  # fit I
              w436 = u16 4  # fit U
              w443 = i16 6 ("precision (6)")
              w366 = "\\" ("regular expression")
              n187 = property on="Splitter" class="Splitter"("Position"=22 ("Splitter Position")) -> ()  [unwired: 2 in, 2 out]
              n188 = property on="Tab Control" class="TabCtl (strict)"("Visible"=TRUE) -> ()  [unwired: 2 in, 2 out]
              n189 = property on="data view" class="WFGraph (strict)"("Visible"=FALSE) -> ()  [unwired: 2 in, 2 out]
              n190 = property on="ln(I,I-bestfit)" class="XYGraph (strict)"() -> ("CrsrList"=w420:T21)  [unwired: 2 in, 2 out]
              n191 = local read "data cut"() -> (w426:T12)
              n192 = control-ref of="VI-fitgraph"() -> (w358:refnum<vi>)
              n193 = case shown="True" "show result" {
                selector: "show result" -> [w542 _]
                frame False {
                  n194 = property on="TeNe" class="XYGraph (strict)"("Visible"=w542) -> ()  [unwired: 2 in, 2 out]
                  n195 = property on="X" class="DigNum (strict)"("Visible"=w542) -> ()  [unwired: 2 in, 2 out]
                  n196 = property on="Y" class="DigNum (strict)"("Visible"=w542) -> ()  [unwired: 2 in, 2 out]
                  n197 = property on="result table" class="Arr (strict)"("Visible"=w542) -> ()  [unwired: 2 in, 2 out]
                  n198 = Not(x=w542) -> (.not. x?=w543:bool)
                  n199 = property on="VI-fitgraph" class="XYGraph (strict)"("Visible"=w543) -> ()  [unwired: 2 in, 2 out]
                  n200 = property on="ln(I,I-bestfit)" class="XYGraph (strict)"("Visible"=w543) -> ()  [unwired: 2 in, 2 out]
                }
                frame True {
                  n201 = local read "TeNe result"() -> (w546:path)
                  n202 = call <vilib>:"Check if File or Folder Exists.vi"("path"=w546) -> ("file or folder exists?"=w544:bool, "dup path"=w545:path)  [unwired: 8 in, 1 out]
                  n203 = case shown="True" w544 {
                    selector: w544 -> [_ w560]
                    tunnel: w545 -> [_ w571]
                    frame False {
                      n204 = One Button Dialog(message="there are no data,\npush \"fit now!\" button\nand than \"write to file\"", button name ("OK")="I see") -> (true=w550:bool)
                      n205 = Not(x=w550) -> (.not. x?=w549:bool)
                      n206 = property on="show result" class="Bool (strict)"("Value"=w549) -> ()  [unwired: 2 in, 2 out]
                    }
                    frame True {
                      w553 = FALSE ("use system decimal point (T)")
                      n207 = property on="TeNe" class="XYGraph (strict)"("Visible"=w560) -> ()  [unwired: 2 in, 2 out]
                      n208 = property on="result table" class="Arr (strict)"("Visible"=FALSE) -> ()  [unwired: 2 in, 2 out]
                      n209 = Not(x=w560) -> (.not. x?=w552:bool)
                      n210 = call-poly <vilib>:"Read From Spreadsheet File.vi"("delimiter (\\t)"="," ("delimiter (\\t)"), "file path (dialog if empty)"=w571) -> ("all rows"=w562:string[][])  [unwired: 5 in, 4 out]
                      "result table" <- w562
                      n211 = property on="X" class="DigNum (strict)"("Visible"=w552) -> ()  [unwired: 2 in, 2 out]
                      n212 = property on="Y" class="DigNum (strict)"("Visible"=w552) -> ()  [unwired: 2 in, 2 out]
                      n213 = property on="VI-fitgraph" class="XYGraph (strict)"("Visible"=w552) -> ()  [unwired: 2 in, 2 out]
                      n214 = property on="ln(I,I-bestfit)" class="XYGraph (strict)"("Visible"=w552) -> ()  [unwired: 2 in, 2 out]
                      n215 = Array Subset(array=w562, index (row)=1 ("index")) -> (w557:string[][])  [unwired: 3 in]
                      n216 = Index Array(array=w557, index (col)=6 ("disabled index (col)")) -> (element=w566:string[])  [unwired: 1 in]
                      n217 = Index Array(array=w557, index (col)=3 ("disabled index (col)")) -> (element=w568:string[])  [unwired: 1 in]
                      n218 = Index Array(array=w557, index (col)=7 ("disabled index (col)")) -> (element=w558:string[])  [unwired: 1 in]
                      n219 = Fract/Exp String To Number(use system decimal point (T)=w553, string=w566) -> (number=w565:dbl[])  [unwired: 2 in, 1 out]
                      n220 = Fract/Exp String To Number(use system decimal point (T)=w553, string=w558) -> (number=w555:dbl[])  [unwired: 2 in, 1 out]
                      n221 = Fract/Exp String To Number(use system decimal point (T)=w553, string=w568) -> (number=w556:dbl[])  [unwired: 2 in, 1 out]
                      n222 = Re/Im To Complex(1:w565, 2:w556) -> (0:w564:cdb[])
                      n223 = Re/Im To Complex(1:w555, 2:w556) -> (0:w554:cdb[])
                      n224 = Build Cluster Array(w564, w554) -> (→"TeNe":cluster{cdb[]}[])
                    }
                  }
                }
              }
              n225 = Unbundle By Name(w426) -> ("data offset array"=w371:dbl[], "data cut array"=w375:waveform(dbl)[], "data lables"=w435:string[])
              n226 = Index Array(array=w420, index=0) -> (element=w422:T15)
              n227 = Unbundle By Name(w422) -> ("Position"=w423:cluster{"X":dbl, "Y":dbl})
              n228 = case shown="False" "Fit scales" {
                tunnel: w358 -> [w449 w457]
                frame False {
                  n229 = case shown="False" "autoscale" {
                    tunnel: w449 -> [w451 w456]
                    frame False {
                      w452 = u8 0 ("X Scale.Scale Fit")
                      w453 = 0 ("Active X Scale")
                      n230 = property class="XYGraph (strict)"(reference=w451, "ActXScl"=w453, "ActYScl"=w453, "XScale.ScaleFit"=w452, "YScale.ScaleFit"=w452) -> ()  [unwired: 1 in, 2 out]
                    }
                    frame True {
                      w454 = u8 2 ("X Scale.Scale Fit")
                      w455 = 0 ("Active X Scale")
                      n231 = property class="XYGraph (strict)"(reference=w456, "ActXScl"=w455, "ActYScl"=w455, "XScale.ScaleFit"=w454, "YScale.ScaleFit"=w454) -> ()  [unwired: 1 in, 2 out]
                    }
                  }
                }
                frame True {
                  w458 = u8 1 ("X Scale.Scale Fit")
                  w459 = 0 ("Active X Scale")
                  n232 = property class="XYGraph (strict)"(reference=w457, "ActXScl"=w459, "ActYScl"=w459, "XScale.ScaleFit"=w458, "YScale.ScaleFit"=w458) -> ()  [unwired: 1 in, 2 out]
                }
              }
              n233 = Index Array "U(volts)shift"(array=w371, index=w436) -> (element=w372:dbl)
              n234 = Index Array "I(A)shift"(array=w371, index=w437) -> (element=w370:dbl)
              n235 = Index Array "U(Volts)"(array=w375, index=w436) -> (element=w376:waveform(dbl))
              n236 = Index Array "to path"(array=w435, index=w437) -> (element=w386:string)
              n237 = Index Array "I(A)"(array=w375, index=w437) -> (element=w427:waveform(dbl))
              n238 = local read "X axis"() -> (w373:u16)
              n239 = Unbundle By Name(w423) -> ("X"=→"X":dbl, "Y"=→"Y":dbl)
              n240 = Reverse String(1:w386) -> (0:w384:string)
              n241 = Get Waveform Attribute(5:T2 {"data path"="", "ADCintercadr_s"=1.0, "data info"={"use or not *.info.txt?"=0, "probe name"="NaN", "signal type"="NaN", "Unit"="NaN", "variable"="NaN", "attenuation factor"=1.0, "amplification factor"=1.0, "extracoef#1"=1.0, "extracoef#2"=1.0, "U cascade, kV"="NaN", "probe area, cm2"=1.0, "plasma, a.m.u."=1.0}, "channel_name"="", "channels_in_file"=0} ("data info template"), 6:"info" ("name"), 7:w427) -> (1:w430:T2, 3:w428:waveform(dbl))  [unwired: 1 in, 2 out]
              n242 = call "waveform-to-XY (SubVI).vi"("waveform"=w376, "offset of cut"=w372, "cut x-axis format"=w373) -> ("Y"=w360:dbl[])  [unwired: 1 out]
              n243 = Match Pattern(string=w384, regular expression=w366) -> (before substring=w385:string, after substring=w387:string)  [unwired: 1 in, 2 out]
              n244 = call "waveform-to-XY (SubVI).vi"("waveform"=w428, "offset of cut"=w370, "cut x-axis format"=w373) -> ("Y"=w359:dbl[])  [unwired: 1 out]
              n245 = Match Pattern(string=w387, regular expression=w366) -> (before substring=w388:string)  [unwired: 1 in, 3 out]
              n246 = Reverse String(1:w385) -> (0:w398:string)
              n247 = Reverse String(1:w387) -> (0:w367:string)
              n248 = Reverse String(1:w388) -> (0:w365:string)
              n249 = Match Pattern(string=w398, regular expression="#") -> (before substring=w408:string)  [unwired: 1 in, 3 out]
              n250 = Concatenate Strings(w367, w366, w365, "_TeNe.txt") -> (w368:string)
              n251 = Match Pattern(string=w408, regular expression="=") -> (before substring=→"TeNe file":string, after substring=→"TeNe interval":string)  [unwired: 1 in, 2 out]
              n252 = String To Path(string=w368) -> (path=→"TeNe result":path)
              n253 = case shown="True" "man.XY table" {
                selector: "man.XY table" -> [w461 _]
                tunnel: [w462 w489] -> w356
                tunnel: [w463 w488] -> w355
                tunnel: w360 -> [w463 _]
                tunnel: w359 -> [w462 _]
                frame False {
                  w460 = T22."Enabled" ("Disabled")
                  n254 = property on="manual I-V input" class="Tbl (strict)"("Visible"=w461) -> ()  [unwired: 2 in, 2 out]
                  n255 = property on="manual I-V source" class="Tbl (strict)"("Visible"=w461) -> ()  [unwired: 2 in, 2 out]
                  n256 = property on="saw bias., V" class="DigNum (strict)"("DisabledEnum"=w460) -> ()  [unwired: 2 in, 2 out]
                  n257 = property on="saw bias., V(ADC)" class="DigNum (strict)"("DisabledEnum"=w460) -> ()  [unwired: 2 in, 2 out]
                }
                frame True {
                  w464 = T22."Disabled and Grayed Out" ("Disabled")
                  w465 = 1.0 ("Value")
                  w466 = "_V-I-manually.txt" ("string")
                  w471 = "\\" ("regular expression")
                  n258 = control-ref of="source"() -> (w478:refnum<vi>)
                  n259 = property class="Clust (strict)"(reference=w478) -> ("Value"=w479:T11)  [unwired: 1 in, 2 out]
                  n260 = property on="manual I-V source" class="Tbl (strict)"("Visible"="show/hide table") -> ()  [unwired: 2 in, 2 out]
                  n261 = property on="manual I-V input" class="Tbl (strict)"("Visible"="show/hide table") -> ()  [unwired: 2 in, 2 out]
                  n262 = Unbundle By Name(w479) -> ("data path"=w473:string[])
                  n263 = Index Array "to path"(array=w473) -> (element=w469:string)  [unwired: 1 in]
                  n264 = Reverse String(1:w469) -> (0:w470:string)
                  n265 = property on="saw bias., V" class="DigNum (strict)"("Value"=w465, "DisabledEnum"=w464) -> ()  [unwired: 2 in, 2 out]
                  n266 = property on="saw bias., V(ADC)" class="DigNum (strict)"("Value"=w465, "DisabledEnum"=w464) -> ()  [unwired: 2 in, 2 out]
                  n267 = Match Pattern(string=w470, regular expression=w471) -> (after substring=w476:string)  [unwired: 1 in, 3 out]
                  n268 = Match Pattern(string=w476, regular expression=w471) -> ()  [unwired: 1 in, 4 out]
                  n269 = Reverse String(1:w476) -> (0:w475:string)
                  n270 = Concatenate Strings(w475, w471, w466) -> (w472:string)
                  n271 = String To Path(string=w472) -> (path=w474:path)
                  n272 = call <vilib>:"Check if File or Folder Exists.vi"("path"=w474) -> ("file or folder exists?"=w467:bool, "dup path"=w468:path)  [unwired: 8 in, 1 out]
                  n273 = case shown="False" w467 {
                    tunnel: w468 -> [_ w504]
                    tunnel: [w496 w505] -> w477
                    tunnel: w466 -> [w493 _]
                    frame False {
                      n274 = call "File Dialog"("prompt"="open file named \"_V-I-manually.txt\",\n located in a folder with proper date", "default name"=w493, "pattern (all files)"="*.txt") -> ("selected path"=w495:path, "cancelled"=w491:bool)  [unwired: 9 in, 2 out]
                      n275 = Strip Path(path=w495) -> (name=w494:string)  [unwired: 1 out]
                      n276 = Not Equal?(x=w494, y=w493) -> (x != y?=w492:bool)
                      n277 = Or(x=w492, y=w491) -> (x .or. y?=w490:bool)
                      n278 = case shown="True" w490 {
                        selector: w490 -> [_ w503]
                        tunnel: w495 -> [w500 _]
                        tunnel: [w499 _] -> w496
                        frame False {
                          n279 = call-poly <vilib>:"Read From Spreadsheet File.vi"("file path (dialog if empty)"=w500) -> ("all rows"=w499:string[][])  [unwired: 6 in, 4 out]
                        }
                        frame True {
                          n280 = call "Display Message to User"("Enable"=w503) -> ("OK"=w502:bool)  [unwired: 9 in, 1 out]
                          n281 = Not(x=w502) -> (.not. x?=w501:bool)
                          n282 = property on="man.XY table" class="Bool (strict)"("Value"=w501) -> ()  [unwired: 2 in, 2 out]
                        }
                      }
                    }
                    frame True {
                      n283 = call-poly <vilib>:"Read From Spreadsheet File.vi"("file path (dialog if empty)"=w504) -> ("all rows"=w505:string[][])  [unwired: 6 in, 4 out]
                    }
                  }
                  "manual I-V source" <- w477
                  n284 = Index Array(array="manual I-V input", index (col)=0 ("index (row)")) -> (element=w484:string[])  [unwired: 1 in]
                  n285 = Index Array(array="manual I-V input", index (col)=1 ("index (row)")) -> (element=w487:string[])  [unwired: 1 in]
                  n286 = Fract/Exp String To Number(use system decimal point (T)=FALSE, string=w484) -> (number=w488:dbl[])  [unwired: 2 in, 1 out]
                  n287 = Fract/Exp String To Number(use system decimal point (T)=FALSE, string=w487) -> (number=w489:dbl[])  [unwired: 2 in, 1 out]
                }
              }
              n288 = Unbundle By Name(w430) -> ("data info"=w431:T19)
              n289 = Unbundle By Name(w431) -> ("probe name"=w446:string, "variable"=w444:string, "probe area, cm2"=w441:dbl, "plasma, a.m.u."=w440:dbl)
              n290 = case shown="True" "manual coef. input" {
                tunnel: w355 -> [w524 w541]
                tunnel: w356 -> [w523 w525]
                tunnel: [w524 w540] -> w353
                tunnel: [w523 w530] -> w352
                tunnel: [w522 w539] -> w439
                tunnel: w440 -> [w522 _]
                tunnel: w441 -> [w521 _]
                tunnel: [w521 w538] -> w442
                tunnel: [w520 w535] -> w445
                tunnel: w444 -> [w520 _]
                tunnel: w446 -> [w519 _]
                tunnel: [w519 w534] -> w447
                frame False {
                  n291 = local read "saw biasing,adc"() -> (w518:dbl)
                  n292 = Absolute Value(x=w518) -> (abs(x)=w517:dbl)
                  n293 = property on="saw bias., V(ADC)" class="DigNum (strict)"("Value"=w517) -> ()  [unwired: 2 in, 2 out]
                }
                frame True {
                  n294 = Unbundle By Name("manual param. input") -> ("R, ohm"=w529:dbl, "I amplif."=w526:dbl, "saw bias., V"=w528:dbl, "saw bias., V(ADC)"=w527:dbl, "plasma, a.u.m."=w539:dbl, "probe area, cm^2"=w538:dbl, "position, etc."=w536:dbl, "probe name"=w534:string)
                  n295 = Divide(x=w528, y=w527) -> (x/y=w532:dbl)
                  n296 = Divide(x=w525, y=w529) -> (x/y=w531:dbl[])
                  n297 = Number To Fractional String(number=w536, precision (6)=i16 6) -> (F-format string=w535:string)  [unwired: 2 in]
                  n298 = Multiply(x=w541, y=w532) -> (x*y=w540:dbl[])
                  n299 = Divide(x=w531, y=w526) -> (x/y=w530:dbl[])
                }
              }
              n300 = local read "param.        manual.     auto?      auto             result"() -> (w412:T10)
              n301 = Index Array(array=w412, index=2) -> (element=w383:T23)
              n302 = Unbundle By Name "Te(eV)"(w383) -> ("result"=w402:dbl)
              n303 = Reciprocal(x=w439) -> (1/x=w390:dbl)
              n304 = Index Array(array=w412, index=0) -> (element=w379:T23)
              n305 = case shown="True" "man. points" {
                tunnel: [w507 w512] -> w354
                tunnel: w353 -> [w507 _]
                tunnel: [w506 w511] -> w357
                tunnel: w352 -> [w506 _]
                frame False {
                }
                frame True {
                  n306 = property on="VI-fitgraph" class="XYGraph (strict)"() -> ("CrsrList"=w510:T21)  [unwired: 2 in, 2 out]
                  n307 = Array Subset(array=w510, index=2) -> (w508:T21)  [unwired: 1 in]
                  n308 = for {
                    tunnel: w508 -> [w516] mode=indexing
                    tunnel: [w514] -> w512 mode=indexing
                    tunnel: [w513] -> w511 mode=indexing
                    n309 = Unbundle By Name(w516) -> ("Position"=w515:cluster{"X":dbl, "Y":dbl})
                    n310 = Unbundle By Name(w515) -> ("X"=w514:dbl, "Y"=w513:dbl)
                  }
                }
              }
              n311 = Unbundle By Name "Is(mA)"(w379) -> ("result"=w401:dbl)
              n312 = Square Root(x=w402) -> (sqrt(x)=w392:dbl)
              n313 = Square Root(x=w390) -> (sqrt(x)=w391:dbl)
              n314 = Divide(x=w401, y=w392) -> (x/y=w394:dbl)
              n315 = Multiply(x=w442, y=w391) -> (x*y=w393:dbl)
              n316 = Index Array(array=w412, index=1) -> (element=w381:T23)
              n317 = Unbundle By Name "Vfl(Volts)"(w381) -> ("result"=w403:dbl)
              n318 = Divide(x=w394, y=w393) -> (x/y=w395:dbl)
              n319 = Multiply(x=9000000000.0, y=w395) -> (x*y=w400:dbl)
              "density, cm^(-3)" <- w400
              n320 = Number To Fractional String "Vfl(Volts)"(use system decimal point (T)=FALSE, number=w403, precision (6)=w443) -> (F-format string=w405:string)  [unwired: 1 in]
              n321 = Number To Fractional String "Is(mA)"(use system decimal point (T)=FALSE, number=w401, precision (6)=w443) -> (F-format string=w404:string)  [unwired: 1 in]
              n322 = Number To Fractional String "Te(eV)"(use system decimal point (T)=FALSE, number=w402, precision (6)=w443) -> (F-format string=w406:string)  [unwired: 1 in]
              n323 = Number To Exponential String(number=w400, precision (6)=w443, 1:FALSE ("use system decimal point (T)")) -> (E-format string=w407:string)  [unwired: 1 in]
              n324 = case shown="True" "save result" {
                tunnel: w447 -> [_ w588]
                tunnel: w445 -> [_ w587]
                tunnel: w404 -> [_ w586]
                tunnel: w405 -> [_ w585]
                tunnel: w406 -> [_ w584]
                tunnel: w407 -> [_ w578]
                frame False {
                }
                frame True {
                  n325 = local read "TeNe result"() -> (w575:path)
                  n326 = local read "TeNe interval"() -> (w576:string)
                  n327 = local read "TeNe file"() -> (w577:string)
                  n328 = call <vilib>:"Check if File or Folder Exists.vi"("path"=w575) -> ("file or folder exists?"=w574:bool, "dup path"=w573:path)  [unwired: 8 in, 1 out]
                  n329 = case shown="False" w574 {
                    tunnel: w573 -> [w590 w604]
                    tunnel: [w589 w604] -> w572
                    frame False {
                      n330 = Build Array("file", "interval", "probe name", "variable", "Is (mA)", "Vfl (Volts)", "Te (eV)", "density (cm**-3)") -> (w596:string[])
                      n331 = Array To Spreadsheet String(delimiter (Tab)=",", array=w596, 3:"%25s" ("format string")) -> (spreadsheet string=w592:string)
                      n332 = call <vilib>:"Write Spreadsheet String.vi"("append to file? (new file:F)"=FALSE ("transpose? (no:F)"), "spreadsheet string"=w592, "file path (dialog if empty)"=w590) -> ("path"=w589:path)  [unwired: 7 in, 1 out]
                    }
                    frame True {
                    }
                  }
                  n333 = Build Array(w577, w576, w588, w587, w586, w585, w584, w578) -> (w582:string[])
                  n334 = Array To Spreadsheet String(delimiter (Tab)=",", array=w582, 3:"%25s" ("format string")) -> (spreadsheet string=w579:string)
                  n335 = call <vilib>:"Write Spreadsheet String.vi"("append to file? (new file:F)"=TRUE ("transpose? (no:F)"), "spreadsheet string"=w579, "file path (dialog if empty)"=w572) -> ()  [unwired: 7 in, 2 out]
                }
              }
              n336 = call "XY sorter (SubVI).vi"("I (A)"=w357, "V (Volt)"=w354) -> ("sorted I (A)"=w361:dbl[], "sorted V (Volt)"=w362:dbl[])  [unwired: 8 in]
              n337 = case shown="False" "processing" {
                tunnel: w361 -> [w617 w636]
                tunnel: w362 -> [w618 w637]
                tunnel: [w625 w638] -> w418
                tunnel: [w619 w634] -> w419
                frame False {
                  n338 = Re/Im To Complex "XY"(1:w617, 2:w618) -> (0:w620:cdb[])
                  n339 = Array Max & Min(array=w618) -> (max value=w611:dbl, min value=w610:dbl)  [unwired: 2 out]
                  n340 = Array Max & Min(array=w617) -> (max value=w613:dbl, min value=w605:dbl)  [unwired: 2 out]
                  n341 = Subtract(x=w611, y=w610) -> (x-y=w614:dbl)
                  n342 = Subtract(x=w613, y=w605) -> (x-y=w612:dbl)
                  n343 = Subtract(x=w613, y=w617) -> (x-y=w623:dbl[])
                  n344 = Build Cluster Array(w620) -> (w625:cluster{cdb[]}[])
                  n345 = Reciprocal(x=w623) -> (1/x=w622:dbl[])
                  n346 = Divide(x=w614, y=2.0) -> (x/y=w609:dbl)
                  n347 = Divide(x=w612, y=2.0) -> (x/y=w606:dbl)
                  n348 = Add(x=w609, y=w610) -> (x+y=w608:dbl)
                  n349 = Add(x=w606, y=w605) -> (x+y=w607:dbl)
                  n350 = Natural Logarithm(1:w622) -> (0:w624:dbl[])
                  n351 = property on="Vf_guess" class="DigNum (strict)"("Value"=w608) -> ()  [unwired: 2 in, 2 out]
                  n352 = property on="Is_guess" class="DigNum (strict)"("Value"=w607) -> ()  [unwired: 2 in, 2 out]
                  n353 = Re/Im To Complex(1:w624, 2:w618) -> (0:w621:cdb[])
                  n354 = Build Cluster Array "ln(I,I-bestfit)"(w621) -> (w619:cluster{cdb[]}[])
                }
                frame True {
                  n355 = control-ref of="VI-fitgraph"() -> (w633:refnum<vi>)
                  n356 = call "Fit.I-V.subvi.vi"("y"=w636, "x"=w637, "Name      Guess     Fit?"="parameter                 manual            auto?", 3:"Parameter Name      Parameter Guess        Fit?"="Parameter Name      Parameter Guess        Fit? 3", 4:"Parameter Name      Parameter Guess        Fit?"="Parameter Name      Parameter Guess        Fit?", "reference"=w633, "set the range by \ncursors?"="Limited by cursors") -> ("parameter guess Fit? best fit result"=w635:T10, "V-I&guess&bestfit"=w632:cluster{cdb[]}[], "ln(I,I-bestfit)"=w634:cluster{cdb[]}[], "error out"=w628:errorcluster)
                  "param.        manual.     auto?      auto             result" <- w635
                  n357 = Unbundle By Name(w628) -> ("status"=w626:bool)
                  n358 = Index Array(array=w635, index=1) -> (element=w647:T23)
                  n359 = Unbundle By Name "Vfl(Volts)"(w647) -> ("result"=w648:dbl)
                  n360 = Not(x=w626) -> (.not. x?=w627:bool)
                  n361 = property on="processing" class="Bool (strict)"("Value"=w627) -> ()  [unwired: 2 in, 2 out]
                  n362 = Re/Im To Complex(1:0.0, 2:w648) -> (0:w644:cdb)
                  n363 = Build Array(w644) -> (w640:cdb[])
                  n364 = Build Cluster Array(w640) -> (w639:cluster{cdb[]}[])
                  n365 = Delete From Array(array=w632, index=1) -> (array with subset deleted=w630:cluster{cdb[]}[])  [unwired: 1 in, 1 out]
                  n366 = Build Array (concatenate)(w630, w639) -> (w638:cluster{cdb[]}[])
                }
              }
              "VI-fitgraph" <- w418
              "ln(I,I-bestfit)" <- w419
            }
            frame #1 {
              n367 = event shown="[0] \"VI-fitgraph\": Mouse Down" {
                selector: _ -> [_ _]
                dyn-events: _ -> [_ _]
                timeout: 200 -> [_ _]
                event "VI-fitgraph": Mouse Down {
                  n368 = event-data() -> ("Coords"=w652:T24, "PlatMods"=w651:T25)  [unwired: 1 in, 6 out]
                  n369 = Unbundle By Name(w651) -> ("Ctrl"=w650:bool)
                  n370 = case shown="True" w650 {
                    tunnel: w652 -> [_ w655]
                    frame False {
                    }
                    frame True {
                      w665 = 0 ("X Scale")
                      n371 = invoke on="VI-fitgraph" class="XYGraph (strict)" method="Map Coords To XY"("Coords"=w655, "X Scale"=w665, "Y Scale"=w665) -> ("XY"=w657:cluster{"X":dbl, "Y":dbl})  [unwired: 4 in, 6 out]
                      n372 = Bundle By Name(cluster=T15 {"Name"="", "Color"=0, "Style"=0, "Point Style"=0, "Name Visible"=FALSE, "Allow Drag"=FALSE, "Cursor Mode"=0, "Plot"=0, "Index"=0, "Position"={"X"=0.0, "Y"=0.0}, "X Scale"=0, "Y Scale"=0, "Watch Plots"=[], "Watch All Plots"=FALSE, "Plot Area"=0, "Label Offset"={"X"=0.0, "Y"=0.0}} ("element"), "Cursor Mode"=u32 0, "Name Visible"="show XY", "Style"=u8 4, "Point Style"=u8 4, "Position"=w657, "Allow Drag"=TRUE, "Color"=u32 14430464) -> (w662:T15)
                      n373 = property on="VI-fitgraph" class="XYGraph (strict)"() -> ("CrsrList"=w664:T21)  [unwired: 2 in, 2 out]
                      n374 = Build Array (concatenate)(w664, w662) -> (w658:T21)
                      n375 = property on="VI-fitgraph" class="XYGraph (strict)"("CrsrList"=w658) -> ()  [unwired: 2 in, 2 out]
                    }
                  }
                }
                event Timeout {
                  n376 = event-data() -> ()  [unwired: 1 in, 3 out]
                }
              }
            }
            frame #2 {
              n377 = control-ref of="VI-fitgraph"() -> (w667:refnum<vi>)
              n378 = case shown="True" "del. points" {
                tunnel: w667 -> [w668 _]
                frame False {
                  n379 = property on="Property Node" class="XYGraph (strict)"(reference=w668) -> (reference out=w670:refnum<vi>, "CrsrList"=w671:T21)  [unwired: 1 in, 1 out]
                  n380 = for {
                    tunnel: w671 -> [w682] mode=indexing
                    tunnel: [w672] -> w669 mode=indexing
                    n381 = Unbundle By Name(w682) -> ("Position"=w674:cluster{"X":dbl, "Y":dbl})
                    n382 = Unbundle By Name(w674) -> ("X"=w680:dbl, "Y"=w676:dbl)
                    n383 = Number To Fractional String(use system decimal point (T)=FALSE, number=w680) -> (F-format string=w679:string)  [unwired: 2 in]
                    n384 = Number To Fractional String(use system decimal point (T)=FALSE, number=w676) -> (F-format string=w675:string)  [unwired: 2 in]
                    n385 = Concatenate Strings(w679, "\n" ("string"), w675) -> (w673:string)
                    n386 = Bundle By Name(cluster=w682, "Name"=w673) -> (w672:T15)
                  }
                  n387 = property on="Property Node" class="XYGraph (strict)"(reference=w670, "CrsrList"=w669) -> ()  [unwired: 1 in, 2 out]
                }
                frame True {
                  n388 = property on="VI-fitgraph" class="XYGraph (strict)"() -> ("CrsrList"=w686:T21)  [unwired: 2 in, 2 out]
                  n389 = Array Size(array=w686) -> (size(s)=w685:i32)
                  n390 = Greater?(x=w685, y=2) -> (0:w683:bool)
                  n391 = case shown="True" w683 {
                    tunnel: w686 -> [_ w693]
                    frame False {
                    }
                    frame True {
                      n392 = Delete From Array(array=w693, length=2, index=0) -> (deleted portion=w687:T21, array with subset deleted=w690:T21)
                      n393 = property on="VI-fitgraph" class="XYGraph (strict)"("CrsrList"=w687) -> ()  [unwired: 2 in, 2 out]
                      n394 = Delete From Array(array=w690, length=1) -> (array with subset deleted=w689:T21)  [unwired: 1 in, 1 out]
                      n395 = Build Array (concatenate)(w687, w689) -> ()  [unwired: 1 out]
                    }
                  }
                }
              }
            }
          }
        }
      }
      n396 = case shown="True" "stop 2" {
        selector: "stop 2" -> [_ w22]
        tunnel: [FALSE w22] -> w14
        frame False {
        }
        frame True {
          n397 = invoke on="data select" class="Clust (strict)" method="Reinit To Default"() -> ()  [unwired: 3 in, 3 out]
        }
      }
      n398 = Equal?(x=w12, y=1) -> (x = y?=w10:bool)
      n399 = case shown="True" w10 {
        tunnel: w9 -> [_ w19]
        frame False {
        }
        frame True {
          n400 = property on="Property Node" class="WFGraph (strict)"(reference=w19, "ActPaletteTool"=u8 5 ("X Scale.Scale Fit")) -> ()  [unwired: 1 in, 2 out]
        }
      }
      n401 = Quit LabVIEW(quit? (T)=w14) -> ()
    }
  }
